vi "Find Item Locations by Path.vi"(5 "Insertion point if not found":bool, 6 "Only return first found":bool, 7 "Path":string, 8 "error in (no error)":errorcluster, 10 "Offset":i32, 11 "JSON":string) -> (0 "error out":errorcluster, 1 "Items":T1[](array[typedef]))   [LabVIEW 2019, in "JSONtext.lvlib"]
uses:
  JSONtext.lvlib
  Parsing/Found Items.ctl
  Parsing/Parsing State.ctl
  Parsing/Advance past Line Ending.vi
  JDP Science Common Utilities/Trim Whitespace__JDP.vi
  Parsing/Advance past whitespace and comma.vi
  Parsing/Advance past next JSON Value (inlined COPY).vi
  Parsing/Advance past Item Name.vi
  Parsing/Advance past next JSON Scaler.vi
  Parsing/Match Pattern.vi
  support/Quote and Escape JSON string.vi
  Parsing/Advance past String.vi
  String Subset.vi
  Parsing/Advance past Number.vi
  support/quote and escape json string 2.vi
  Parsing/Advance past Array.vi
  Parsing/Advance past Object.vi
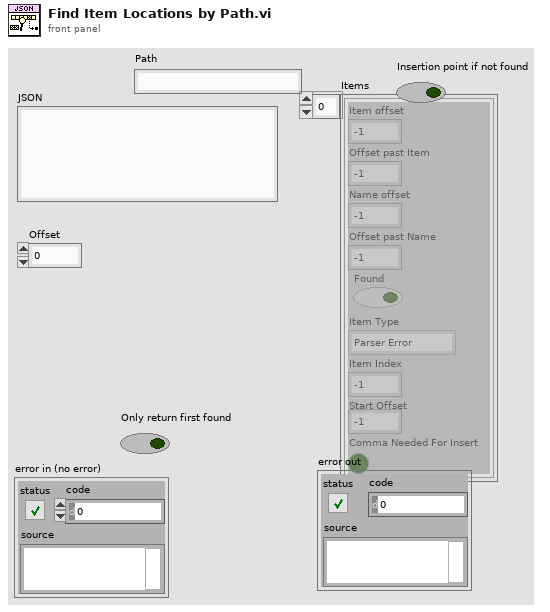
[diagram p1: front panel]
types:
  T1 = typedef "JSONtext.lvlib/Found Items.ctl" = cluster{"Item offset":i32, "Offset past Item":i32, "Name offset":i32, "Offset past Name":i32, "Found":bool, "Item Type":T2, "Item Index":i32, "Start Offset":i32, "Comma Needed For Insert":bool}
  T2 = typedef "JSONtext.lvlib/Parsing State.ctl" = enum16{"Parser Error", "Object", "Array", "String", "Number/Other", "Leading Whitespace", "Object end", "Array end", "Value end"}
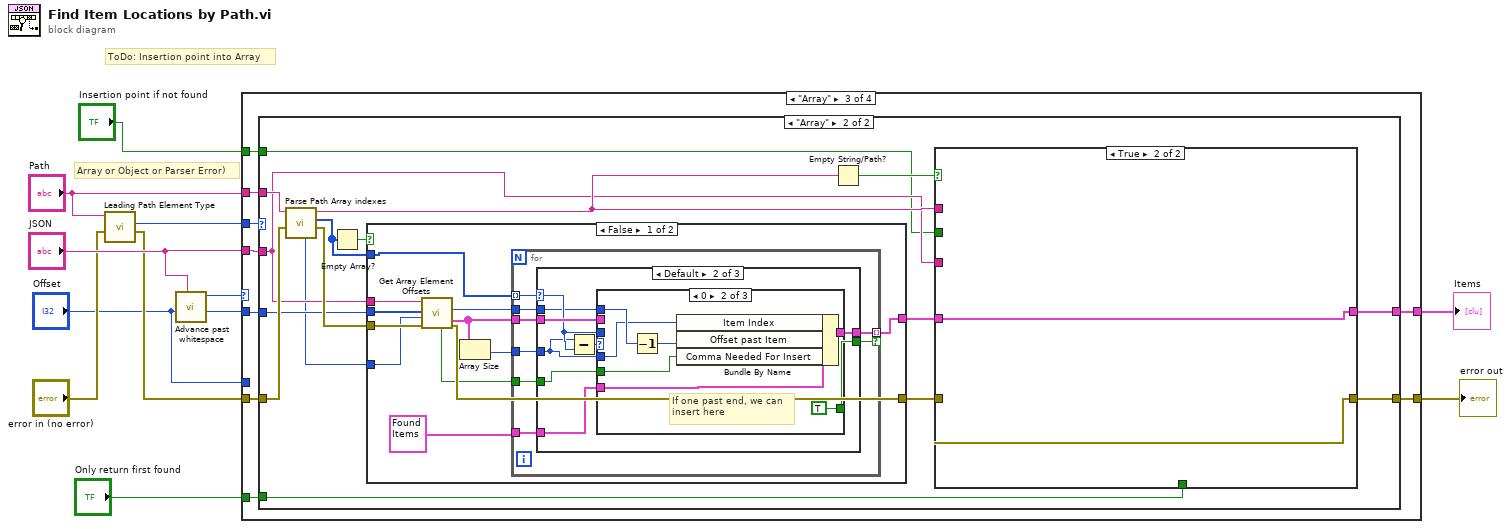
[diagram p0: block diagram]
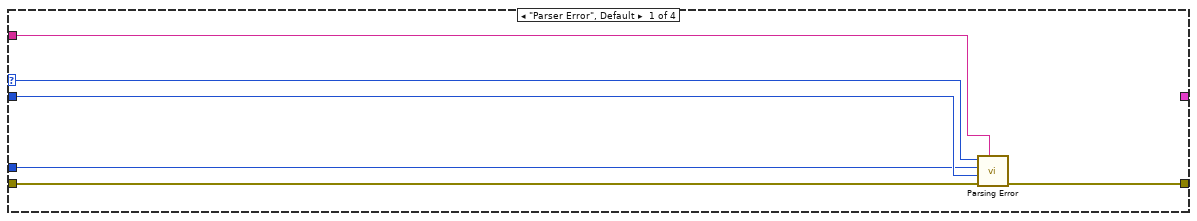
[diagram p2: hidden frame]
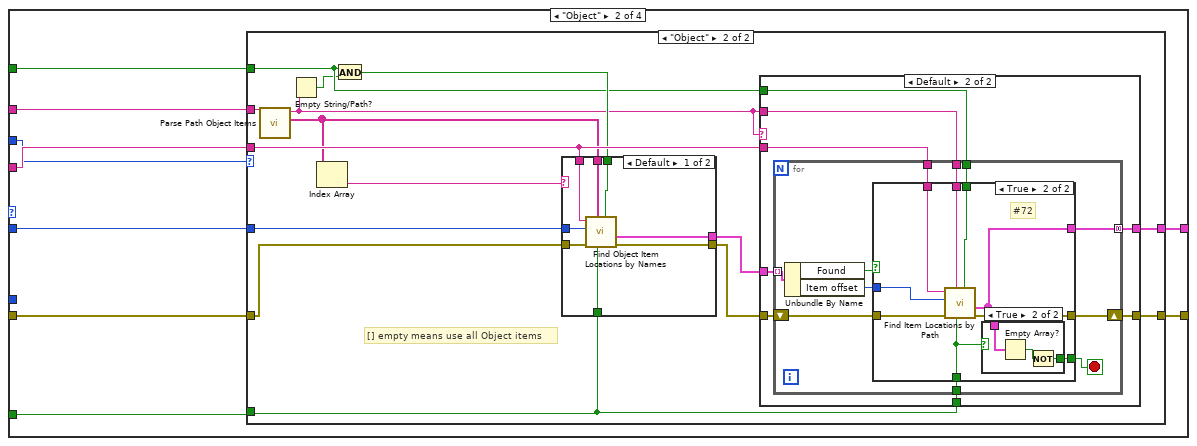
[diagram p3: hidden frame]
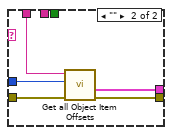
[diagram p5: hidden frame]
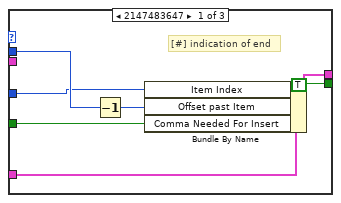
[diagram p10: hidden frame]
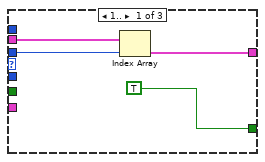
[diagram p11: hidden frame]
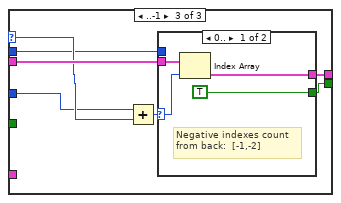
[diagram p13: hidden frame]
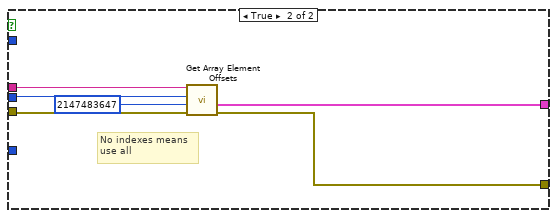
[diagram p15: hidden frame]
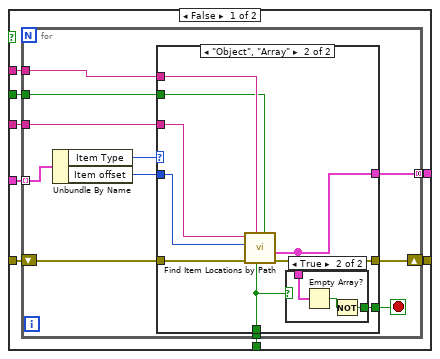
[diagram p16: hidden frame]
diagram:
  # "Array or Object or Parser Error)"
  # "ToDo: Insertion point into Array"
  n1 = call "Leading Path Element Type.vi"("error in (no error)"="error in (no error)", "Path"="Path") -> ("error out"=w4:errorcluster, "Path Element Type (Array or Object or Parser Error)"=w1:T2)  [unwired: 8 in]
  n2 = call "Advance past whitespace.vi"("JSON"="JSON", "Offset"="Offset") -> ("Offset of first non-whitespace"=w10:i32, "Parser State"=w3:T2)  [unwired: 7 in, 1 out]
  n3 = case shown="\"Array\"" w3 {
    selector: w3 -> [w16 _ _ _]
    tunnel: [_ w26 w98 _] -> w12
    tunnel: w4 -> [w18 w24 w95 w215]
    tunnel: [w17 w27 w99 w215] -> w9
    tunnel: "Path" -> [_ w23 w96 _]
    tunnel: "Only return first found" -> [_ w21 w97 _]
    tunnel: "Insertion point if not found" -> [_ w20 w91 _]
    tunnel: w10 -> [w15 w22 w94 _]
    tunnel: "JSON" -> [w14 w25 w93 _]
    tunnel: "Offset" -> [w13 _ _ _]
    tunnel: w1 -> [_ w19 w92 _]
    frame "Parser Error", Default {
      n4 = call "Parsing Error.vi"("JSON"=w14, "error in (no error)"=w18, "Offset past match"=w15, "Value start"=w13, "State"=w16) -> ("error out"=w17:errorcluster)  [unwired: 6 in]
    }
    frame "Object" {
      n5 = case shown="\"Object\"" w19 {
        tunnel: [w28 w43] -> w27
        tunnel: [_ w42] -> w26
        tunnel: w25 -> [_ w41]
        tunnel: w24 -> [w28 w40]
        tunnel: w23 -> [_ w39]
        tunnel: w22 -> [_ w38]
        tunnel: w21 -> [_ w33]
        tunnel: w20 -> [_ w31]
        frame Default {
        }
        frame "Object" {
          # "[] empty means use all Object items"
          n6 = call "Parse Path Object Items.vi"("Path with leading Object element"=w39) -> ("<JSON>items names"=w35:string[], "Rest or Path"=w29:string)  [unwired: 7 in, 2 out]
          n7 = Empty String/Path?(string/path=w29) -> (empty?=w30:bool)
          n8 = Index Array(array=w35) -> (element=w34:string)  [unwired: 1 in]
          n9 = And(x=w31, y=w30) -> (x .and. y?=w32:bool)
          n10 = case shown="Default" w34 {
            tunnel: w41 -> [w51 w56]
            tunnel: w40 -> [w50 w54]
            tunnel: w38 -> [w49 w55]
            tunnel: w35 -> [w48 _]
            tunnel: [w47 w53] -> w37
            tunnel: [w46 w52] -> w36
            tunnel: w33 -> [w45 _]
            tunnel: w32 -> [w44 _]
            frame Default {
              n11 = call "Find Object Item Locations by Names.vi"("Insertion point if not found"=w44, "Only return first found"=w45, "Item Names <JSON>"=w48, "error in (no error)"=w50, "Object Offset"=w49, "JSON"=w51) -> ("error out"=w47:errorcluster, "Items"=w46:T1[])  [unwired: 4 in]
            }
            frame "" {
              n12 = call "Get all Object Item Offsets.vi"("error in (no error)"=w54, "Offset"=w55, "JSON"=w56) -> ("error out"=w53:errorcluster, "Items"=w52:T1[])  [unwired: 6 in, 1 out]
            }
          }
          n13 = case shown="Default" w29 {
            tunnel: [w57 w66] -> w43
            tunnel: [w58 w65] -> w42
            tunnel: w41 -> [_ w64]
            tunnel: w29 -> [_ w63]
            tunnel: w37 -> [w57 w62]
            tunnel: w36 -> [w58 w61]
            tunnel: w33 -> [_ w60]
            tunnel: w31 -> [_ w59]
            frame "" {
            }
            frame Default {
              n14 = for {
                tunnel: [w76] -> w65 mode=concatenating
                tunnel: w64 -> [w75]
                tunnel: w63 -> [w74]
                tunnel: w61 -> [w72] mode=indexing
                shift-right: [w77] -> w66
                shift-left: w62 -> [w73]
                tunnel: w60 -> [w69]
                tunnel: w59 -> [w67]
                stop <- w68 stop-if-true
                n15 = Unbundle By Name(w72) -> ("Found"=w71:bool, "Item offset"=w70:i32)
                n16 = case shown="True" w71 {
                  tunnel: [w78 w87] -> w77
                  tunnel: [_ w81] -> w76
                  tunnel: w75 -> [_ w86]
                  tunnel: w74 -> [_ w85]
                  tunnel: w73 -> [w78 w84]
                  tunnel: w70 -> [_ w83]
                  tunnel: w69 -> [_ w82]
                  tunnel: [_ w80] -> w68
                  tunnel: w67 -> [_ w79]
                  frame False {
                  }
                  frame True {
                    # "#72"
                    n17 = call "Find Item Locations by Path.vi"("Insertion point if not found"=w79, "Only return first found"=w82, "Path"=w85, "error in (no error)"=w84, "Offset"=w83, "JSON"=w86) -> ("error out"=w87:errorcluster, "Items"=w81:T1[])  [unwired: 4 in]
                    n18 = case shown="True" w82 {
                      tunnel: w81 -> [_ w90]
                      tunnel: [_ w88] -> w80
                      frame False {
                      }
                      frame True {
                        n19 = Empty Array?(array=w90) -> (empty?=w89:bool)
                        n20 = Not(x=w89) -> (.not. x?=w88:bool)
                      }
                    }
                  }
                }
              }
            }
          }
        }
      }
    }
    frame "Array" {
      n21 = case shown="\"Array\"" w92 {
        tunnel: [w100 w116] -> w99
        tunnel: [_ w115] -> w98
        tunnel: w97 -> [_ w114]
        tunnel: w96 -> [_ w113]
        tunnel: w95 -> [w100 w112]
        tunnel: w94 -> [_ w105]
        tunnel: w93 -> [_ w104]
        tunnel: w91 -> [_ w101]
        frame "Parser Error", Default {
        }
        frame "Array" {
          n22 = call "Parse Path Array indexes.vi"("error in (no error)"=w112, "Path with leading Array element"=w113) -> ("error out"=w106:errorcluster, "Indexes (empty means use all)"=w107:i32[], "Rest or Path"=w111:string, "Max Index to parse"=w102:i32)  [unwired: 6 in]
          n23 = Empty Array?(array=w107) -> (empty?=w109:bool)
          n24 = case shown="False" w109 {
            tunnel: [w128 w176] -> w108
            tunnel: w107 -> [w120 _]
            tunnel: w106 -> [w126 w178]
            tunnel: w105 -> [w125 w179]
            tunnel: w104 -> [w124 w180]
            tunnel: [w123 w177] -> w103
            tunnel: w102 -> [w119 _]
            frame False {
              n25 = call "Get Array Element Offsets.vi"("error in (no error)"=w126, "Max Index"=w119, "Offset"=w125, "JSON"=w124) -> ("error out"=w123:errorcluster, "Elements"=w122:T1[], "Offset past Array"=w121:i32, "Comma Needed for Insert"=w117:bool)  [unwired: 4 in]
              n26 = Array Size(array=w122) -> (size(s)=w127:i32)
              n27 = for {
                tunnel: w120 -> [w134] mode=indexing
                tunnel: w122 -> [w136]
                tunnel: [w135] -> w128 mode=indexing if=w131
                tunnel: w127 -> [w133]
                tunnel: w121 -> [w132]
                tunnel: T1 {"Item offset"=0, "Offset past Item"=0, "Name offset"=-1, "Offset past Name"=-1, "Found"=FALSE, "Item Type"=enum."Parser Error", "Item Index"=0, "Start Offset"=-1, "Comma Needed For Insert"=FALSE} -> [w130]
                tunnel: w117 -> [w129]
                n28 = case shown="Default" w134 {
                  selector: w134 -> [_ w150 w168]
                  tunnel: w136 -> [_ w152 w170]
                  tunnel: [w143 w151 w169] -> w135
                  tunnel: w133 -> [w139 w146 w164]
                  tunnel: [TRUE w149 w167] -> w131
                  tunnel: w132 -> [w142 w147 w165]
                  tunnel: w130 -> [w138 w145 _]
                  tunnel: w129 -> [w137 w144 _]
                  frame 2147483647 {
                    # "[#] indication of end"
                    n29 = Decrement(x=w142) -> (x-1=w141:i32)
                    n30 = Bundle By Name(cluster=w138, "Item Index"=w139, "Offset past Item"=w141, "Comma Needed For Insert"=w137) -> (w143:T1)
                  }
                  frame Default {
                    n31 = Subtract(x=w146, y=w150) -> (x-y=w148:i32)
                    n32 = case shown="0" w148 {
                      tunnel: w152 -> [w156 _ _]
                      tunnel: [w155 w161 _] -> w151
                      tunnel: w150 -> [w154 _ _]
                      tunnel: [TRUE TRUE _] -> w149
                      tunnel: w147 -> [_ w160 _]
                      tunnel: w146 -> [_ w158 _]
                      tunnel: w145 -> [_ w159 _]
                      tunnel: w144 -> [_ w157 _]
                      frame 1.. {
                        n33 = Index Array(array=w156, index=w154) -> (element=w155:T1)
                      }
                      frame 0 {
                        # "If one past end, we can\ninsert here"
                        n34 = Decrement(x=w160) -> (x-1=w163:i32)
                        n35 = Bundle By Name(cluster=w159, "Item Index"=w158, "Offset past Item"=w163, "Comma Needed For Insert"=w157) -> (w161:T1)
                      }
                      frame Default {
                      }
                    }
                  }
                  frame ..-1 {
                    n36 = Add(x=w164, y=w168) -> (x+y=w166:i32)
                    n37 = case shown="0.." w166 {
                      selector: w166 -> [w171 _]
                      tunnel: w170 -> [w174 _]
                      tunnel: [w173 _] -> w169
                      tunnel: [TRUE _] -> w167
                      tunnel: w165 -> [_ _]
                      frame 0.. {
                        # "Negative indexes count\nfrom back:  [-1,-2]"
                        n38 = Index Array(array=w174, index=w171) -> (element=w173:T1)
                      }
                      frame Default {
                      }
                    }
                  }
                }
              }
            }
            frame True {
              # "No indexes means\nuse all"
              n39 = call "Get Array Element Offsets.vi"("error in (no error)"=w178, "Max Index"=2147483647, "Offset"=w179, "JSON"=w180) -> ("error out"=w177:errorcluster, "Elements"=w176:T1[])  [unwired: 4 in, 2 out]
            }
          }
          n40 = Empty String/Path?(string/path=w111) -> (empty?=w110:bool)
          n41 = case shown="True" w110 {
            tunnel: [w188 w214] -> w116
            tunnel: [w187 w213] -> w115
            tunnel: w108 -> [w186 w213]
            tunnel: w103 -> [w185 w214]
            tunnel: w104 -> [w184 _]
            tunnel: w114 -> [w183 _]
            tunnel: w111 -> [w182 _]
            tunnel: w101 -> [w181 _]
            frame False {
              n42 = for {
                tunnel: [w197] -> w187 mode=concatenating
                shift-right: [w198] -> w188
                shift-left: w185 -> [w199]
                tunnel: w182 -> [w196]
                tunnel: w186 -> [w195] mode=indexing
                tunnel: w184 -> [w193]
                tunnel: w183 -> [w191]
                tunnel: w181 -> [w189]
                stop <- w190 stop-if-true
                n43 = Unbundle By Name(w195) -> ("Item Type"=w194:T2, "Item offset"=w192:i32)
                n44 = case shown="\"Object\", \"Array\"" w194 {
                  tunnel: w199 -> [w200 w209]
                  tunnel: [w200 w208] -> w198
                  tunnel: [_ w204] -> w197
                  tunnel: w196 -> [_ w207]
                  tunnel: w193 -> [_ w206]
                  tunnel: w192 -> [_ w205]
                  tunnel: w191 -> [_ w202]
                  tunnel: [_ w203] -> w190
                  tunnel: w189 -> [_ w201]
                  frame "Parser Error", Default {
                  }
                  frame "Object", "Array" {
                    n45 = call "Find Item Locations by Path.vi"("Insertion point if not found"=w201, "Only return first found"=w202, "Path"=w207, "error in (no error)"=w209, "Offset"=w205, "JSON"=w206) -> ("error out"=w208:errorcluster, "Items"=w204:T1[])  [unwired: 4 in]
                    n46 = case shown="True" w202 {
                      tunnel: w204 -> [_ w212]
                      tunnel: [_ w210] -> w203
                      frame False {
                      }
                      frame True {
                        n47 = Empty Array?(array=w212) -> (empty?=w211:bool)
                        n48 = Not(x=w211) -> (.not. x?=w210:bool)
                      }
                    }
                  }
                }
              }
            }
            frame True {
            }
          }
        }
      }
    }
    frame "String", "Number/Other" {
      # "Not an object or Array so Path ends here\n\n--> throw error?"
    }
  }
  "Items" <- w12
  "error out" <- w9
